vi "Hardware_Module_z2.vi"(6 "LEDs":refnum<vi>, 7 "State":enum16{"Configure Port", "Write", "Close"}(ring), 8 "error in (no error)":errorcluster, 9 "write buffer":string, 10 "baud rate (9600)":u32=9600, 11 "VISA resource name":refnum<visa-resource-name>) -> (0 "error out":errorcluster, 2 "return count":u32, 3 "VISA resource name out":refnum<visa-resource-name>)   [LabVIEW 2024]
doc: "Funkcja służy do komunikacji za pomocą portu szeregowergo z modułem EvB5.1, który zawiera mikroporcesor Atmega32. Komunikacja odbywa się poprzez bibliotekę NI-VISA z wykorzystaniem podstawowych funkcji portu szeregowego. Funkcja umożliwia emulację hardwaru i softwaru wówczas jako nazwę urządzenia podać: VirtualDevice1\n\n- VISA resource name specifies the resource to be opened.\n- baud rate is the rate of transmission. The default is 9600. \n- write buffer contains the data to be written to the device. \n- return count contains the actual number of bytes written. \n- State defines the functionality of the function. It contains three values Configure Port, Write and Close\n- LEDs is used during emulation. This is a reference to boolean array.\n- error out contains error information. This output provides standard error out functionality.\n\nWięcej pomocy można znaleźć w pomocy funkcji:\nVISA Configure Serial Port VI \nVISA Write Function"
uses:
  <vilib>/Instr/_visa.llb/VISA Configure Serial Port (Instr).vi
panel:
  # "Inputs"
  # "Outputs"
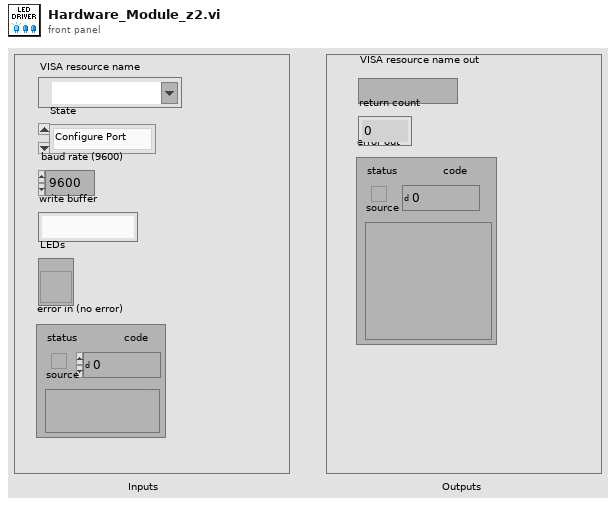
[diagram p1: front panel]
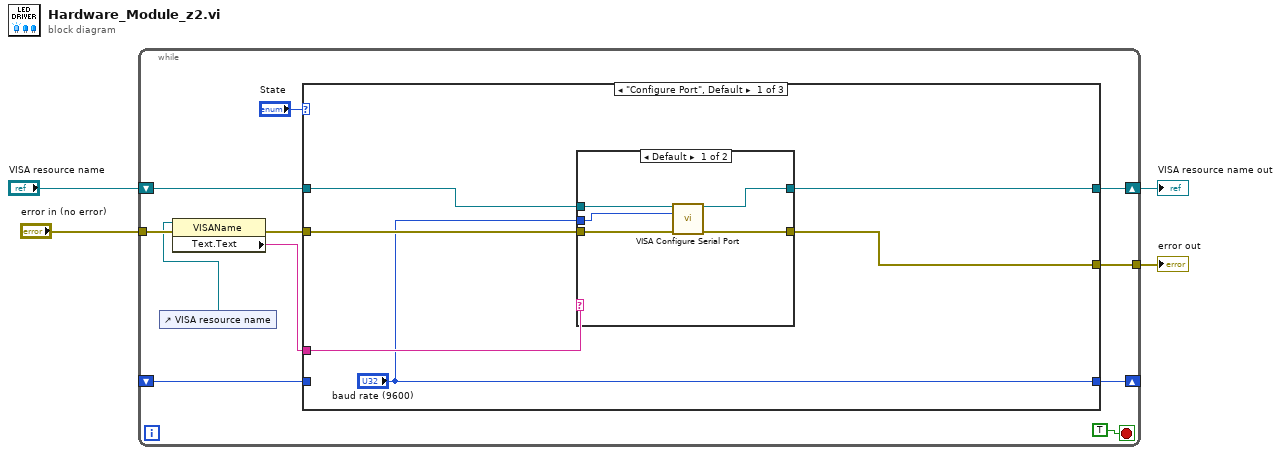
[diagram p0: block diagram]
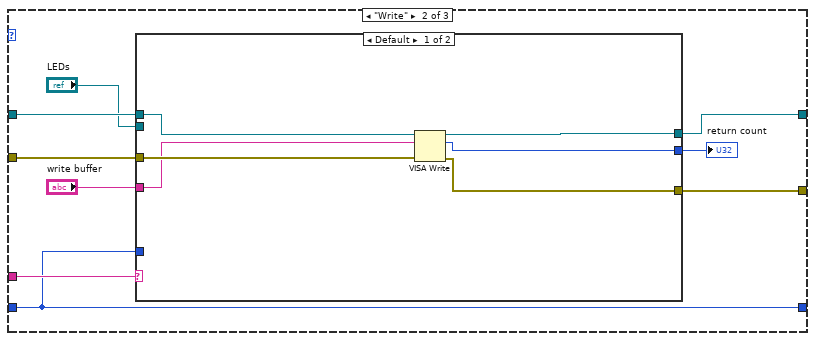
[diagram p3: hidden frame]
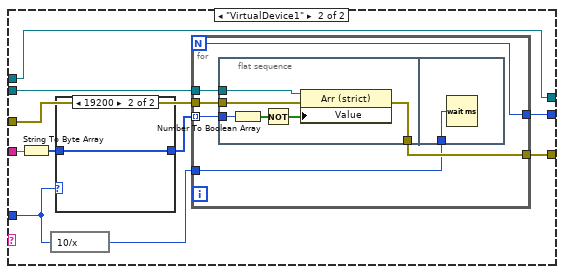
[diagram p4: hidden frame]
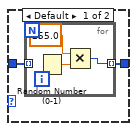
[diagram p5: hidden frame]
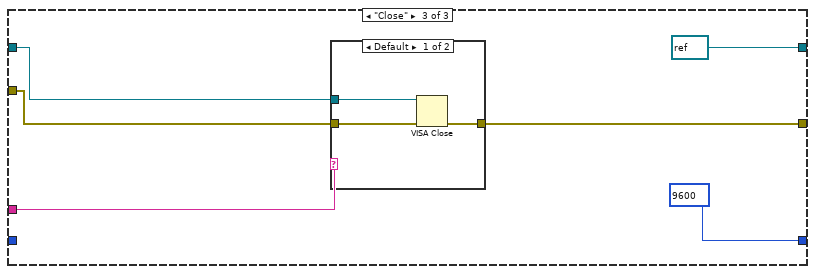
[diagram p6: hidden frame]
diagram:
  n1 = while {
    tunnel: "error in (no error)" -> [w14]
    tunnel: [w12] -> w2
    shift-right: [w13] -> w3
    shift-left: "VISA resource name" -> [w6]
    shift-right: [w10] -> _
    shift-left: _ -> [w7]
    stop <- TRUE stop-if-true
    n2 = control-ref of="VISA resource name"() -> (w5:refnum<vi>)
    n3 = property on="Property Node" class="VISAName"(reference=w5, error in=w14) -> (error out=w9:errorcluster, "Text.Text"=w8:string)  [unwired: 1 out]
    n4 = case shown="\"Configure Port\", Default" "State" {
      tunnel: [w21 w37 refnum<visa-resource-name> refnum ("VISA resource name")] -> w13
      tunnel: [w20 w30 w76] -> w12
      tunnel: w6 -> [w19 w36 w77]
      tunnel: ["baud rate (9600)" w29 u32 9600 ("baud rate (9600)")] -> w10
      tunnel: w9 -> [w18 w34 w74]
      tunnel: w8 -> [w17 w35 w75]
      tunnel: w7 -> [_ w29 _]
      frame "Configure Port", Default {
        n5 = case shown="Default" w17 {
          tunnel: w18 -> [w26 w28]
          tunnel: [w25 w27] -> w21
          tunnel: [w24 w28] -> w20
          tunnel: w19 -> [w23 w27]
          tunnel: "baud rate (9600)" -> [w22 _]
          frame Default {
            n6 = call-poly "VISA Configure Serial Port"("VISA resource name"=w23, "baud rate (9600)"=w22, "error in (no error)"=w26) -> ("VISA resource name out"=w25:refnum<visa-resource-name>, "error out"=w24:errorcluster)  [unwired: 11 in]
          }
          frame "VirtualDevice1" {
          }
        }
      }
      frame "Write" {
        n7 = case shown="Default" w35 {
          tunnel: w36 -> [w43 w52]
          tunnel: [w40 w50] -> w30
          tunnel: w34 -> [w41 w51]
          tunnel: [w42 w52] -> w37
          tunnel: "write buffer" -> [w39 w46]
          tunnel: [w38 w49] -> w32
          tunnel: "LEDs" -> [_ w53]
          tunnel: w29 -> [_ w47]
          frame Default {
            n8 = VISA Write(VISA resource name=w43, write buffer=w39, error in (no error)=w41) -> (VISA resource name out=w42:refnum<visa-resource-name>, return count=w38:u32, error out=w40:errorcluster)
          }
          frame "VirtualDevice1" {
            n9 = String To Byte Array(string=w46) -> (unsigned byte array=w45:u8[])
            n10 = expression code="10/x"(w47) -> (w48:u32)
            n11 = case shown="19200" w47 {
              tunnel: w45 -> [w55 w59]
              tunnel: [w54 w59] -> w44
              frame Default {
                n12 = for {
                  tunnel: w55 -> [_] mode=indexing
                  tunnel: [w57] -> w54 mode=indexing
                  n13 = Random Number (0-1)() -> (number: 0 to 1=w58:dbl)
                  n14 = Multiply(x=255.0, y=w58) -> (x*y=w57:u8)
                }
              }
              frame 19200 {
              }
            }
            n15 = for {
              N -> [w61]
              tunnel: w53 -> [w65]
              tunnel: w44 -> [w62] mode=indexing
              tunnel: w51 -> [w63]
              tunnel: [w64] -> w50
              tunnel: [w61] -> w49
              tunnel: w48 -> [w60]
              n16 = flat-sequence {
                tunnel: w65 -> [w71]
                tunnel: [w70] -> w64
                tunnel: w63 -> [w69]
                tunnel: w62 -> [w68]
                tunnel: w60 -> [w72]
                frame #0 {
                  n17 = Number To Boolean Array(number=w68) -> (Boolean array=w67:bool[])
                  n18 = Not(x=w67) -> (.not. x?=w66:bool[])
                  n19 = property class="Arr (strict)"(reference=w71, error in=w69, "Value"=w66) -> (error out=w70:errorcluster)  [unwired: 1 out]
                }
                frame #1 {
                  n20 = Wait (ms)(milliseconds to wait=w72) -> ()  [unwired: 1 out]
                }
              }
            }
          }
        }
        "return count" <- w32
      }
      frame "Close" {
        n21 = case shown="Default" w75 {
          tunnel: w77 -> [w81 _]
          tunnel: [w80 w82] -> w76
          tunnel: w74 -> [w79 w82]
          frame Default {
            n22 = VISA Close(VISA resource name=w81, error in (no error)=w79) -> (error out=w80:errorcluster)
          }
          frame "VirtualDevice1" {
          }
        }
      }
    }
  }
  "VISA resource name out" <- w3
  "error out" <- w2
